vi "Upload.vi"(7 "ICommunicate":refnum<class "ICommunicate.lvclass">, 8 "Error In":errorcluster, 9 "Multiplexer":cluster{"Index":u16, "Sub-Index":u8} {"Sub-Index" format="%.0x"; "Index" format="%04x"}, 10 "Node-ID":u8, 11 "reference in":refnum<class "SDO Manager.lvclass">) -> (0 "Error Out":errorcluster, 1 "Value":u8[](array[numeric]) format="%.0x", 2 "Success?":bool, 3 "reference out":refnum<class "SDO Manager.lvclass">)   [LabVIEW 2024, in "CANopen Master.lvlib" / "SDO Manager.lvclass"]
uses:
  SDO Manager.lvclass
  SDO Manager.lvclass/SDO Manager.ctl
  CANopen Request/CANopen Request Message.lvclass
  Service Data Object/Service Data Object.lvclass
  CANopen Message/CANopen Message.lvclass
  HAL/Source/Interfaces/ICommunicate/ICommunicate.lvclass
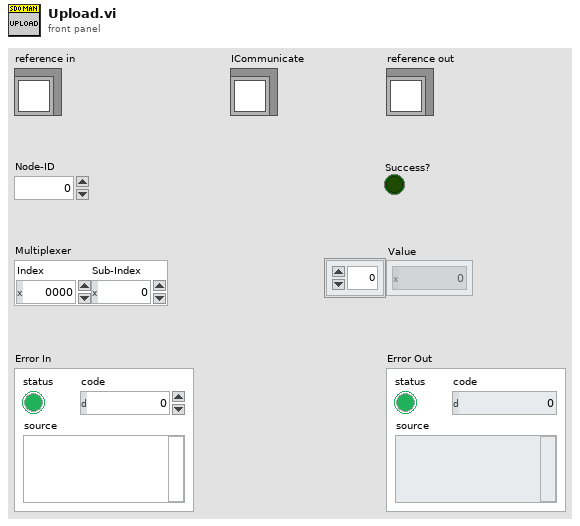
[diagram p1: front panel]
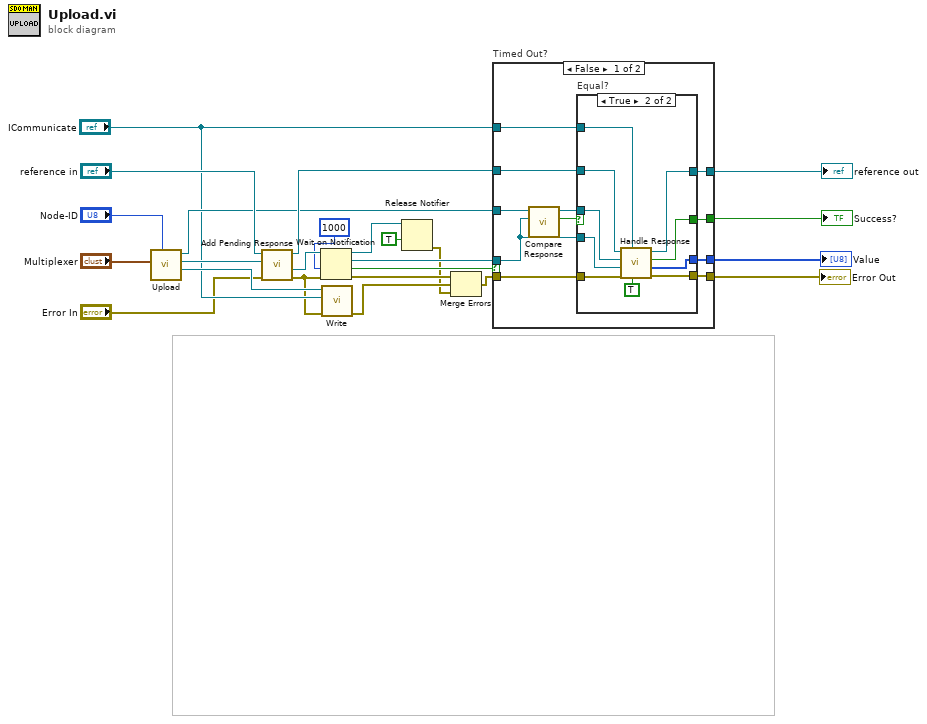
[diagram p0: block diagram]
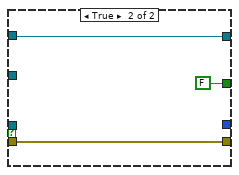
[diagram p3: hidden frame]
diagram:
  n1 = call "Upload.vi"("Node-ID"="Node-ID", "Multiplexer"="Multiplexer") -> ("Request"=w21:refnum<class "CANopen Request Message.lvclass">, "Expected Response"=w20:refnum<class "CANopen Response Message.lvclass">, "Service Data Object out"=w14:refnum<class "Service Data Object.lvclass">)  [unwired: 7 in]
  n2 = call "Add Pending Response.vi"("Error In"="Error In", "Expected Response"=w20, "reference in"="reference in") -> ("Error Out"=w6:errorcluster, "Response Notifier out"=w18:refnum<notifier>, "reference out"=w17:refnum<class "SDO Manager.lvclass">)  [unwired: 6 in]
  n3 = Wait on Notification(notifier=w18, timeout in ms (-1)=1000 ("timeout in ms"), error in (no error)=w6) -> (notifier out=w3:refnum<notifier>, notification=w9:refnum<class "CANopen Response Message.lvclass">, timed out?=w8:bool, error out=w4:errorcluster)  [unwired: 1 in]
  n4 = call "Write.vi"("error in"=w6, "ICommunicate"="ICommunicate", "CANopen Message in"=w21) -> ("error out"=w7:errorcluster)  [unwired: 7 in, 1 out]
  n5 = Release Notifier(notifier=w3, force destroy? (F)=TRUE) -> (error out=w2:errorcluster)  [unwired: 1 in, 2 out]
  n6 = Merge Errors(w4, w7, w2) -> (w5:errorcluster)
  n7 = case "Timed Out?" shown="False" w8 {
    tunnel: w5 -> [w35 w51]
    tunnel: [w31 w51] -> w16
    tunnel: w9 -> [w30 _]
    tunnel: w14 -> [w34 _]
    tunnel: [w26 FALSE ("Equal?")] -> w22
    tunnel: "ICommunicate" -> [w32 _]
    tunnel: w17 -> [w28 w49]
    tunnel: [w27 w49] -> w15
    tunnel: [w25 _] -> w12
    frame False {
      n8 = call "Compare Response.vi"("Actual"=w30, "Service Data Object"=w34) -> ("Equal?"=w33:bool, "Service Data Object out"=w29:refnum<class "Service Data Object.lvclass">)  [unwired: 8 in]
      n9 = case "Equal?" shown="True" w33 {
        selector: w33 -> [w37 _]
        tunnel: w32 -> [_ w44]
        tunnel: w35 -> [w36 w48]
        tunnel: [w36 w47] -> w31
        tunnel: w30 -> [_ w46]
        tunnel: w29 -> [_ w45]
        tunnel: w28 -> [w38 w43]
        tunnel: [w38 w42] -> w27
        tunnel: [w37 w41] -> w26
        tunnel: [_ w40] -> w25
        frame False {
        }
        frame True {
          n10 = call "Handle Response.vi"("Last Toggle-Bit"=TRUE, "ICommunicate"=w44, "Error In"=w48, "Response"=w46, "Service Data Object"=w45, "reference in"=w43) -> ("Error Out"=w47:errorcluster, "Value"=w40:u8[], "Success?"=w41:bool, "reference out"=w42:refnum<class "SDO Manager.lvclass">)  [unwired: 2 in]
        }
      }
    }
    frame True {
    }
  }
  "Error Out" <- w16
  "reference out" <- w15
  "Success?" <- w22
  "Value" <- w12
